vi "Configure Spectrum Emission Mask (Bandwidth Setup).vi"(0 "VISA resource name":refnum<visa-resource-name>, 5 "SEM Auto Resolution Bandwidth (1:On)":i32(ring)=1 items=["Off", "On"], 7 "SEM Resolution Bandwidth (4:3 kHz)":i32(ring)=4 items=["30 Hz", "100 Hz", "300 Hz", "1 kHz", "3 kHz", "10 kHz", "30 kHz", "100 kHz", "300 kHz", "1 MHz", "3 MHz", "50 kHz", "5 MHz", "10 MHz", "20 MHz"], 9 "SEM Auto Video Bandwidth (1:On)":i32(ring)=1 items=["Off", "On"], 11 "error in (no error)":errorcluster, 12 "SEM Video Bandwidth (8:3kHz)":i32(ring)=8 items=["OFF", "1 Hz", "3 Hz", "10 Hz", "30 Hz", "100 Hz", "300 Hz", "1 kHz", "3 kHz", "10 kHz", "30 kHz", "100 kHz", "300 kHz", "1 MHz", "3 MHz", "10 MHz", "5 kHz"], 13 "SEM Video Bandwidth (0:Normal VBW)":i32(ring) items=["Normal VBW", "Power VBW"]) -> (4 "VISA resource name out":refnum<visa-resource-name>, 15 "error out":errorcluster)   [LabVIEW 2020, in "Anritsu Signal Analyzer Series.lvlib"]
doc: "Configures the bandwidth for reference parameter of SEM measurement settings of the spectrum analyzer."
uses:
  Anritsu Signal Analyzer Series.lvlib
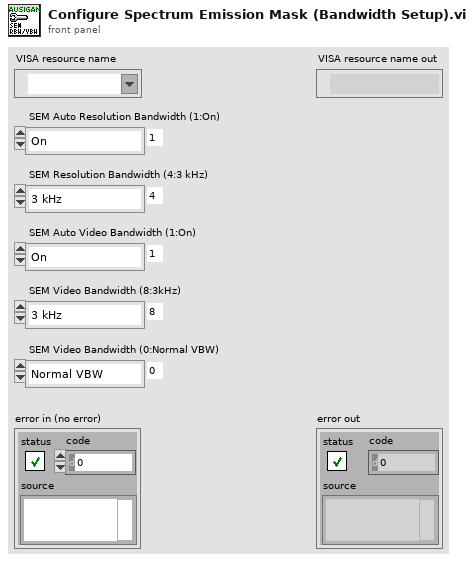
[diagram p1: front panel]
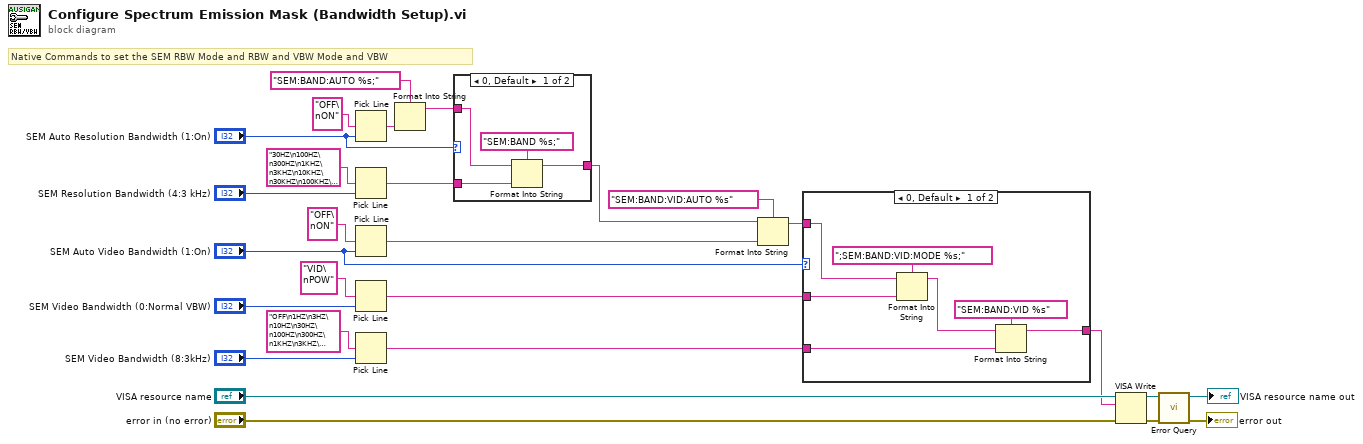
[diagram p0: block diagram]
diagram:
  # "Native Commands to set the SEM RBW Mode and RBW and VBW Mode and VBW"
  n1 = Pick Line(multi-line string="OFF\nON" ("複数行文字列"), line index="SEM Auto Resolution Bandwidth (1:On)") -> (output string=w11:string)  [unwired: 1 in]
  n2 = Pick Line(multi-line string="30HZ\n100HZ\n300HZ\n1KHZ\n3KHZ\n10KHZ\n30KHZ\n100KHZ\n300KHZ\n1MHZ\n3MHZ\n50KHZ\n5MHZ\n10MHZ\n20MHZ" ("複数行文字列"), line index="SEM Resolution Bandwidth (4:3 kHz)") -> (output string=w3:string)  [unwired: 1 in]
  n3 = Pick Line(multi-line string="OFF\nON" ("複数行文字列"), line index="SEM Auto Video Bandwidth (1:On)") -> (output string=w9:string)  [unwired: 1 in]
  n4 = Pick Line(multi-line string="VID\nPOW" ("複数行文字列"), line index="SEM Video Bandwidth (0:Normal VBW)") -> (output string=w7:string)  [unwired: 1 in]
  n5 = Pick Line(multi-line string="OFF\n1HZ\n3HZ\n10HZ\n30HZ\n100HZ\n300HZ\n1KHZ\n3KHZ\n10KHZ\n30KHZ\n100KHZ\n300KHZ\n1MHZ\n3MHZ\n5MHZ\n10MHZ\n5KHZ" ("複数行文字列"), line index="SEM Video Bandwidth (8:3kHz)") -> (output string=w5:string)  [unwired: 1 in]
  n6 = Format Into String(format string="SEM:BAND:AUTO %s;" ("_CommandSet"), w11) -> (resulting string=w16:string)  [unwired: 2 in, 1 out]
  n7 = case shown="0, Default" "SEM Auto Resolution Bandwidth (1:On)" {
    tunnel: w3 -> [w31 _]
    tunnel: w16 -> [w30 w32]
    tunnel: [w28 w32] -> w15
    frame 0, Default {
      n8 = Format Into String(format string="SEM:BAND %s;" ("_CommandSet"), initial string=w30, w31) -> (resulting string=w28:string)  [unwired: 1 in, 1 out]
    }
    frame 1 {
    }
  }
  n9 = Format Into String(format string="SEM:BAND:VID:AUTO %s" ("_CommandSet"), initial string=w15, w9) -> (resulting string=w13:string)  [unwired: 1 in, 1 out]
  n10 = case shown="0, Default" "SEM Auto Video Bandwidth (1:On)" {
    tunnel: w7 -> [w39 _]
    tunnel: w13 -> [w38 w40]
    tunnel: w5 -> [w36 _]
    tunnel: [w33 w40] -> w18
    frame 0, Default {
      n11 = Format Into String(format string=";SEM:BAND:VID:MODE %s;" ("_CommandSet"), initial string=w38, w39) -> (resulting string=w35:string)  [unwired: 1 in, 1 out]
      n12 = Format Into String(format string="SEM:BAND:VID %s" ("_CommandSet"), initial string=w35, w36) -> (resulting string=w33:string)  [unwired: 1 in, 1 out]
    }
    frame 1 {
    }
  }
  n13 = VISA Write(VISA resource name="VISA resource name", write buffer=w18, error in (no error)="error in (no error)") -> (VISA resource name out=w19:refnum<visa-resource-name>, error out=w20:errorcluster)  [unwired: 1 out]
  n14 = call "Error Query.vi"("error in (no error)"=w20, "VISA resource name"=w19) -> ("error out"=→"error out":errorcluster, "VISA resource name out"=→"VISA resource name out":refnum<visa-resource-name>)  [unwired: 6 in, 2 out]
